vi "getStatesFromXML.vi"(8 "error in (no error)":errorcluster, 9 "xmlPath":string, 10 "channel_configXML":refnum<class "NativeXML.lvclass">, 11 "RfOutputChannel in":refnum<class "RfOutputChannel.lvclass">) -> (0 "error out":errorcluster, 2 "channel_configXML":refnum<class "NativeXML.lvclass">, 3 "RfOutputChannel out":refnum<class "RfOutputChannel.lvclass">)   [LabVIEW 2009, in "Tools.lvlib" / "DatabaseHelpers.lvlib" / "RfOutputChannel.lvclass"]
uses:
  RfOutputChannel.lvclass
  NativeXML/NativeXML.lvclass
  RfOutputChannel.lvclass/RfOutputChannel.ctl
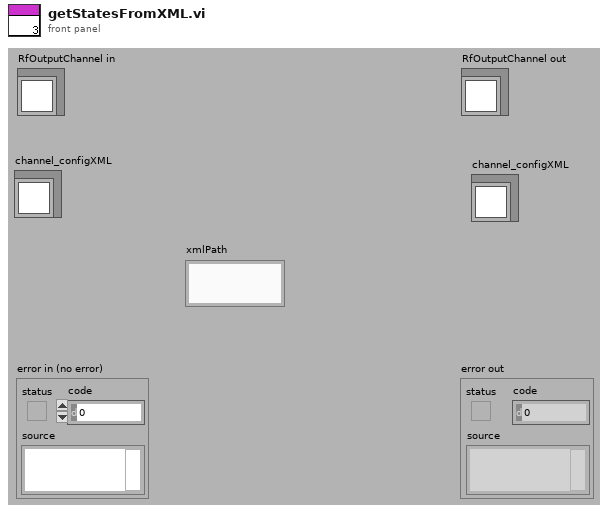
[diagram p1: front panel]
types:
  T1 = cluster{"state_name":string, "value":cluster{"frequency":string, "amplitude":string, "phase":string}}[]
  T2 = cluster{"state_name":string, "value":cluster{"frequency":string, "amplitude":string, "phase":string}}
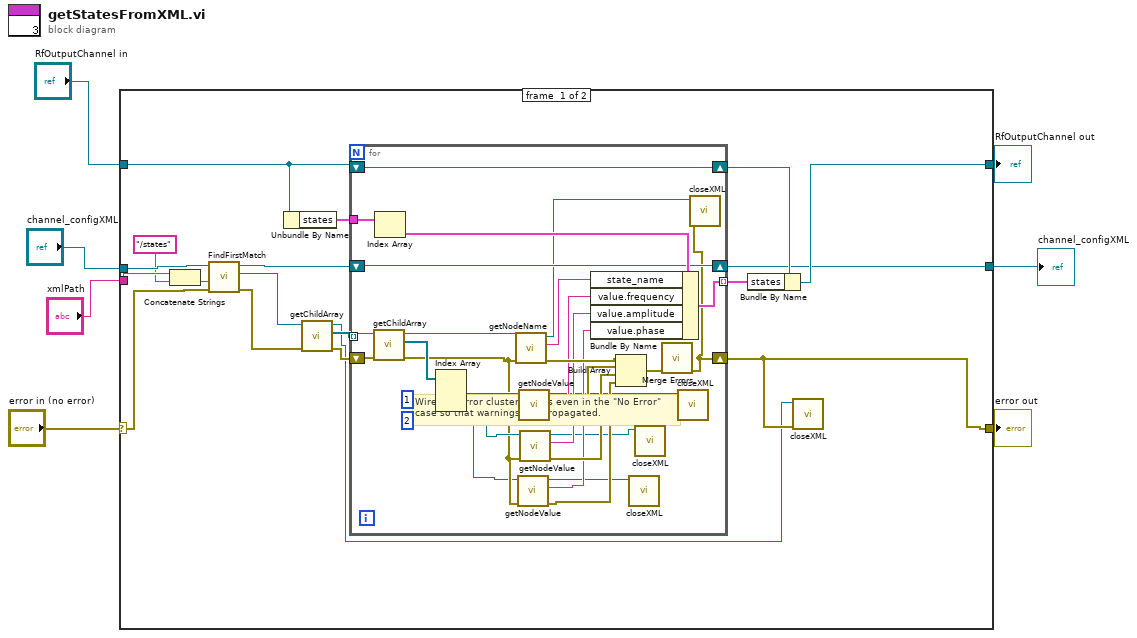
[diagram p0: block diagram]
diagram:
  n1 = case shown="No Error" "error in (no error)" {
    selector: "error in (no error)" -> [w13 w56]
    tunnel: [w17 w56] -> w6
    tunnel: [w21 w55] -> w4
    tunnel: "RfOutputChannel in" -> [w22 w55]
    tunnel: "channel_configXML" -> [w14 _]
    tunnel: [w20 _] -> w2
    tunnel: "xmlPath" -> [w11 _]
    frame #0 {
      # "Wire the error cluster across even in the \"No Error\"\ncase so that warnings get propagated."
      n2 = Concatenate Strings(w11, "/states") -> (w12:string)
      n3 = call "FindFirstMatch.vi"("error in (no error)"=w13, "xPath"=w12, "NativeXML in"=w14) -> ("error out"=w9:errorcluster, "NativeXML match"=w8:refnum<class "NativeXML.lvclass">, "NativeXML out"=w15:refnum<class "NativeXML.lvclass">)  [unwired: 6 in]
      n4 = Unbundle By Name(w22) -> ("states"=w25:T1)
      n5 = call "getChildArray.vi"("error in (no error)"=w9, "NativeXML in"=w8) -> ("error out"=w19:errorcluster, "childArray"=w18:refnum<class "NativeXML.lvclass">[], "NativeXML out"=w16:refnum<class "NativeXML.lvclass">)  [unwired: 7 in]
      n6 = for {
        shift-right: [w26] -> w17
        shift-left: w19 -> [w44]
        tunnel: w18 -> [w46] mode=indexing
        shift-right: [w49] -> w24
        shift-left: w22 -> [w49]
        tunnel: w25 -> [w52]
        tunnel: [w50] -> w23 mode=indexing
        shift-right: [w47] -> w20
        shift-left: w15 -> [w47]
        n7 = call "getChildArray.vi"("error in (no error)"=w44, "NativeXML in"=w46) -> ("error out"=w32:errorcluster, "childArray"=w45:refnum<class "NativeXML.lvclass">[], "NativeXML out"=w42:refnum<class "NativeXML.lvclass">)  [unwired: 7 in]
        n8 = Index Array(array=w52) -> (element=w51:T2)  [unwired: 1 in]
        n9 = Index Array(array=w45, index #2=1, index #3=2) -> (element #1=w38:refnum<class "NativeXML.lvclass">, element #2=w35:refnum<class "NativeXML.lvclass">, element #3=w31:refnum<class "NativeXML.lvclass">)  [unwired: 1 in]
        n10 = call "getNodeName.vi"("error in (no error)"=w32, "NativeXML in"=w42) -> ("error out"=w43:errorcluster, "name"=w41:string, "NativeXML out"=w27:refnum<class "NativeXML.lvclass">)  [unwired: 7 in]
        n11 = call "getNodeValue.vi"("error in (no error)"=w32, "NativeXML in"=w31) -> ("error out"=w34:errorcluster, "Value"=w33:string, "NativeXML out"=w30:refnum<class "NativeXML.lvclass">)  [unwired: 7 in]
        n12 = call "getNodeValue.vi"("NativeXML in"=w38) -> ("error out"=w40:errorcluster, "Value"=w39:string, "NativeXML out"=w28:refnum<class "NativeXML.lvclass">)  [unwired: 8 in]
        n13 = call "getNodeValue.vi"("error in (no error)"=w32, "NativeXML in"=w35) -> ("error out"=w37:errorcluster, "Value"=w36:string, "NativeXML out"=w29:refnum<class "NativeXML.lvclass">)  [unwired: 7 in]
        n14 = Bundle By Name(cluster=w51, "state_name"=w41, "value.frequency"=w39, "value.amplitude"=w36, "value.phase"=w33) -> (w50:T2)
        n15 = Build Array(w43, w40, w37, w34) -> (w48:errorcluster[])
        n16 = call "closeXML.vi"("NativeXML in"=w30) -> ()  [unwired: 10 in, 1 out]
        n17 = call "closeXML.vi"("NativeXML in"=w29) -> ()  [unwired: 10 in, 1 out]
        n18 = call <vilib>:"Merge Errors.vi"("error array in"=w48) -> ("error out"=w26:errorcluster)  [unwired: 6 in]
        n19 = call "closeXML.vi"("NativeXML in"=w28) -> ()  [unwired: 10 in, 1 out]
        n20 = call "closeXML.vi"("error in (no error)"=w26, "NativeXML in"=w27) -> ()  [unwired: 9 in, 1 out]
      }
      n21 = Bundle By Name(cluster=w24, "states"=w23) -> (w21:refnum<class "RfOutputChannel.lvclass">)
      n22 = call "closeXML.vi"("error in (no error)"=w17, "NativeXML in"=w16) -> ()  [unwired: 9 in, 1 out]
    }
    frame #1 {
    }
  }
  "error out" <- w6
  "RfOutputChannel out" <- w4
  "channel_configXML" <- w2
